vi "Mutate_v1_to_v2.vi"(11 "SerializableData_v1":T5) -> (0 "error out":errorcluster, 3 "SerializableData":T1)   [LabVIEW 2019, in "Kobe Bryant.lvclass"]
uses:
  Kobe Bryant.lvclass
  SerializableData_v1.ctl
  SerializableData.ctl
  KobeData1.ctl
  KobeData2.ctl
  KobeEnum.ctl
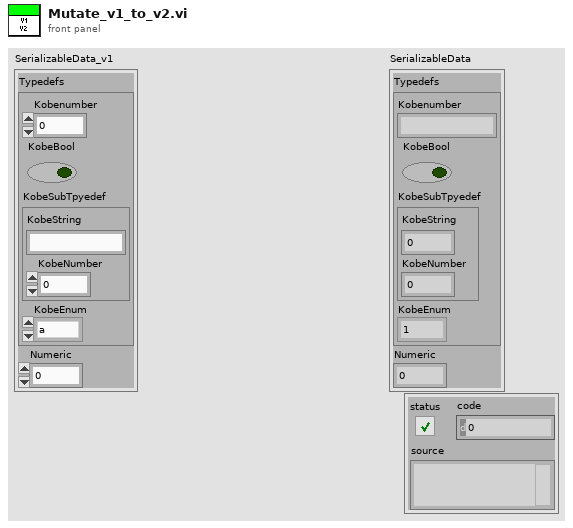
[diagram p1: front panel]
types:
  T1 = typedef "Kobe Bryant.lvclass/SerializableData.ctl" = cluster{"Typedefs":T2, "Numeric":dbl}
  T2 = typedef "Kobe Bryant.lvclass/KobeData1.ctl" = cluster{"Kobenumber":string, "KobeBool":bool, "KobeSubTpyedef":T3, "KobeEnum":T4}
  T3 = typedef "Kobe Bryant.lvclass/KobeData2.ctl" = cluster{"KobeString":dbl, "KobeNumber":dbl}
  T4 = typedef "Kobe Bryant.lvclass/KobeEnum.ctl" = enum16{"1", "2", "3", "4", "5"}
  T5 = typedef "Kobe Bryant.lvclass/SerializableData_v1.ctl" = cluster{"Typedefs":cluster{"Kobenumber":dbl, "KobeBool":bool, "KobeSubTpyedef":cluster{"KobeString":string, "KobeNumber":dbl}, "KobeEnum":enum16{"a", "b", "c", "d", "e"}}, "Numeric":dbl}
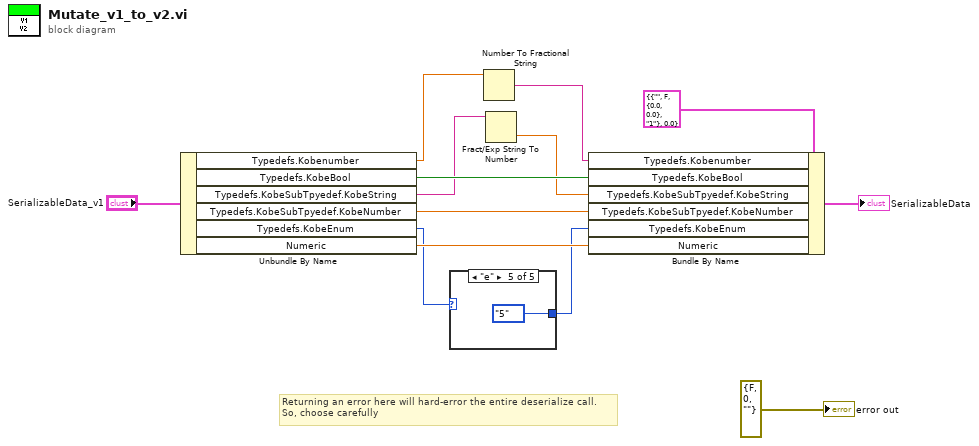
[diagram p0: block diagram]
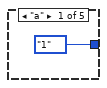
[diagram p2: hidden frame]
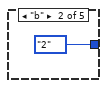
[diagram p3: hidden frame]
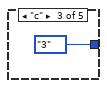
[diagram p4: hidden frame]
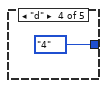
[diagram p5: hidden frame]
diagram:
  # "Returning an error here will hard-error the entire deserialize call.\nSo, choose carefully"
  n1 = Unbundle By Name("SerializableData_v1") -> ("Typedefs.Kobenumber"=w9:dbl, "Typedefs.KobeBool"=w7:bool, "Typedefs.KobeSubTpyedef.KobeString"=w6:string, "Typedefs.KobeSubTpyedef.KobeNumber"=w4:dbl, "Typedefs.KobeEnum"=w2:enum16{"a", "b", "c", "d", "e"}, "Numeric"=w3:dbl)
  n2 = case shown="\"e\"" w2 {
    tunnel: [KobeEnum."1" ("Typedefs.KobeEnum") KobeEnum."2" ("Typedefs.KobeEnum") KobeEnum."3" ("Typedefs.KobeEnum") KobeEnum."4" ("Typedefs.KobeEnum") KobeEnum."5" ("Typedefs.KobeEnum")] -> w1
    frame "a" {
    }
    frame "b" {
    }
    frame "c" {
    }
    frame "d" {
    }
    frame "e" {
    }
  }
  n3 = Number To Fractional String(number=w9) -> (F-format string=w8:string)  [unwired: 3 in]
  n4 = Fract/Exp String To Number(string=w6) -> (number=w5:dbl)  [unwired: 3 in, 1 out]
  n5 = Bundle By Name(cluster=T1 {"Typedefs"={"Kobenumber"="", "KobeBool"=FALSE, "KobeSubTpyedef"={"KobeString"=0.0, "KobeNumber"=0.0}, "KobeEnum"=enum."1"}, "Numeric"=0.0} ("SerializableData"), "Typedefs.Kobenumber"=w8, "Typedefs.KobeBool"=w7, "Typedefs.KobeSubTpyedef.KobeString"=w5, "Typedefs.KobeSubTpyedef.KobeNumber"=w4, "Typedefs.KobeEnum"=w1, "Numeric"=w3) -> (→"SerializableData":T1)
  "error out" <- errorcluster {"status"=FALSE, "code"=0, "source"=""} ("error out")
